vi "SaveFromMemory.vi"(8 "error in (no error)":errorcluster, 10 "Data_2_Save":T1(array[cluster]), 11 "DBAL-SQLite in":refnum<class "DBAL-SQLite.lvclass">) -> (0 "error out":errorcluster, 3 "DBAL-SQLite out":refnum<class "DBAL-SQLite.lvclass">)   [LabVIEW 2020, in "Sgraph_lib_V1.lvlib" / "DBAL-SQLite.lvclass"]
doc: "Must override!"
uses:
  DBAL-SQLite.lvclass
  DBAL.lvclass
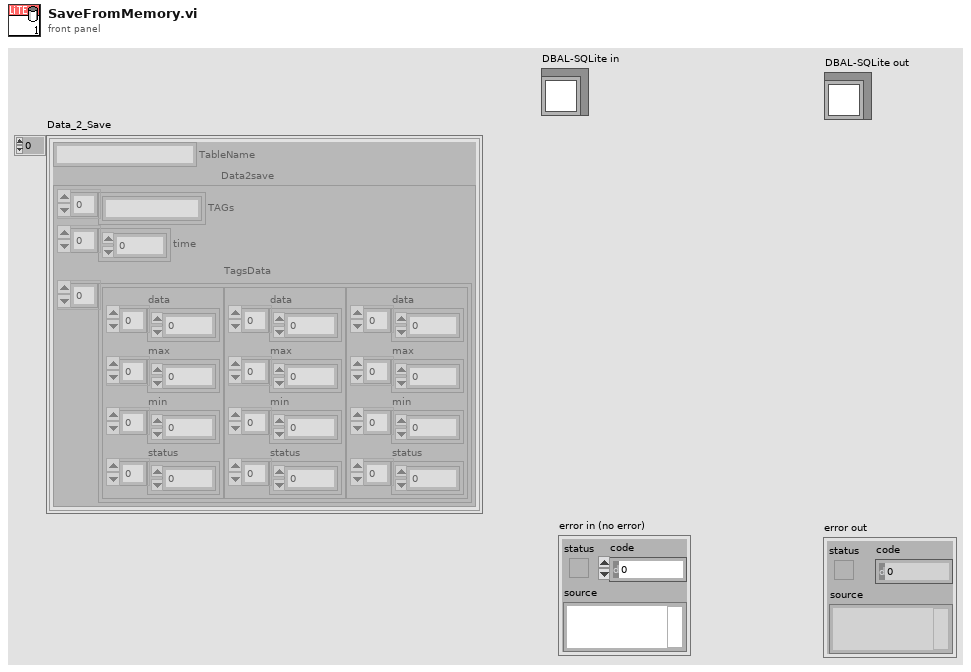
[diagram p1: front panel]
types:
  T1 = cluster{"TableName":string, "Data2save":cluster{"TAGs":string[], "time":dbl[], "TagsData":cluster{"data":dbl[], "max":dbl[], "min":dbl[], "status":u32[]}[]}}[]
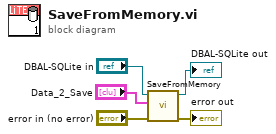
[diagram p0: block diagram]
diagram:
  n1 = call-parent "SaveFromMemory.vi"("error in (no error)"="error in (no error)", "Data_2_Save"="Data_2_Save", "DBAL in"="DBAL-SQLite in") -> ("error out"=→"error out":errorcluster, "DBAL out"=→"DBAL-SQLite out":refnum<class "DBAL-SQLite.lvclass">)  [unwired: 7 in]
